vi "Core Chooser.vi"(11 "online devices":T1[](array[typedef])) -> (3 "selected device":T1)   [LabVIEW 2013, in "Particle API.lvlib"]
uses:
  Particle API.lvlib
  Controls/Device Query JSON.ctl
panel:
  in  "OK Button":bool
  in  "Devices":string(combo)
  # "Multiple Particle devices are available. Please choose which one you would like to connect to:"
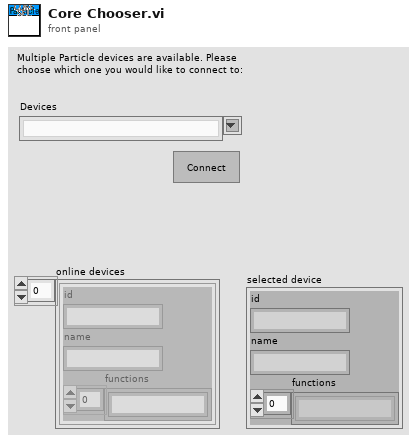
[diagram p1: front panel]
types:
  T1 = typedef "Particle API.lvlib/Device Query JSON.ctl" = cluster{"id":string, "name":string, "functions":string[]}
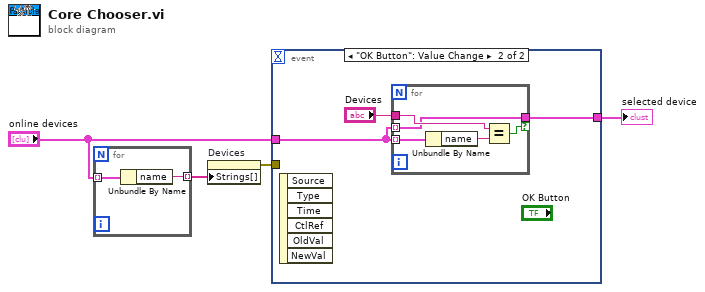
[diagram p0: block diagram]
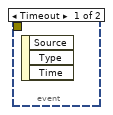
[diagram p2: hidden frame]
diagram:
  n1 = for {
    tunnel: "online devices" -> [w6] mode=indexing
    tunnel: [w5] -> w4 mode=indexing
    n2 = Unbundle By Name(w6) -> ("name"=w5:string)
  }
  n3 = property on="Devices" class="CmbBox"("Strings[]"=w4) -> (error out=w3:errorcluster)  [unwired: 2 in, 1 out]
  n4 = event shown="[1] \"OK Button\": Value Change" {
    selector: _ -> [_ _]
    dyn-events: _ -> [_ _]
    timeout: _ -> [_ _]
    tunnel: w3 -> [_ _]
    tunnel: "online devices" -> [_ w8]
    tunnel: [_ w7] -> w1
    event Timeout {
      n5 = event-data() -> ()  [unwired: 1 in, 3 out]
    }
    event "OK Button": Value Change {
      n6 = event-data() -> ()  [unwired: 1 in, 6 out]
      n7 = for {
        tunnel: w8 -> [w14] mode=indexing
        tunnel: "Devices" -> [w12]
        tunnel: [w10] -> w7 if=w11
        tunnel: w8 -> [w10] mode=indexing
        n8 = Unbundle By Name(w14) -> ("name"=w13:string)
        n9 = Equal?(x=w12, y=w13) -> (x = y?=w11:bool)
      }
    }
  }
  "selected device" <- w1
